vi "Sensor_Camera Auton Simple.vi"(7 "Final Task":T1(ring), 8 "error in":errorcluster, 9 "Second Drive Distance":dbl, 10 "First Turn Angle":dbl, 11 "First Drive Distance":dbl) -> (0 "error out":errorcluster)   [LabVIEW 2016]
uses:
  <vilib>/Rock Robotics/WPI/Gyro/WPI_GyroDevRef.ctl
  <vilib>/Rock Robotics/SystemInterfaces/AI/FPGA_AIChannel.ctl
  <vilib>/Rock Robotics/SystemInterfaces/spilib/spi_bus.ctl
  <vilib>/Rock Robotics/WPI/DriverStation/WPI_DriverStationAllianceInfo.ctl
  Vision/Vision Drive/Vision Drive.lvlib
  SubSystems/Drive/Drive System.lvlib
  SubSystems/Path Track/Path Track.lvlib
  SubSystems/Intake/Intake.lvlib
panel:
  in  "Vision Deadband":dbl=25.0 caption="Vision Deadband Distance (in.)"
  in  "Drive Magnitude":dbl format="%#_13g"
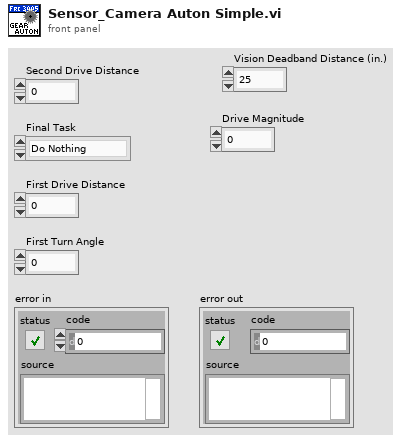
[diagram p1: front panel]
types:
  T1 = enum16{"Do Nothing", "Turn Up Field", "Turn to Boiler"}
  T2 = typedef "WPI_GyroDevRef.ctl" = cluster{"DevStatus":errorcluster, "Analog Channel":T3, "Offset":dbl, "Gain (VoltsPerDegree/Second)":dbl, "Gyro Type":enum16{"Analog", "XRS450"}, "Handle":i32, "SPI Bus":T4, "Device Found":bool, "Sample Rate":dbl, "Calibrate On Open":bool}
  T3 = typedef "FPGA_AIChannel.ctl" = enum8{"AI 0", "AI 1", "AI 2", "AI 3", "AI MXP 0", "AI MXP 1", "AI MXP 2", "AI MXP 3", "Invalid"}
  T4 = typedef "spi_bus.ctl" = enum16{"SPI On-Board, CS0", "SPI On-Board, CS1", "SPI On-Board, CS2", "SPI On-Board, CS3", "SPI MXP", "Invalid"}
  T5 = typedef "WPI_DriverStationAllianceInfo.ctl" = enum16{"Red", "Blue", "Invalid"}
  T6 = cluster{"Gyro":T2, "First Drive Distance":dbl, "First Turn Angle":dbl, "Alliance":T5, "Vision Timeout?":bool, "Vision Distance":dbl, "Second Drive Distance":dbl, "Final Task":enum16{"Do Nothing", "Turn Up Field", "Turn to Boiler"}, "Vision Angle":dbl}
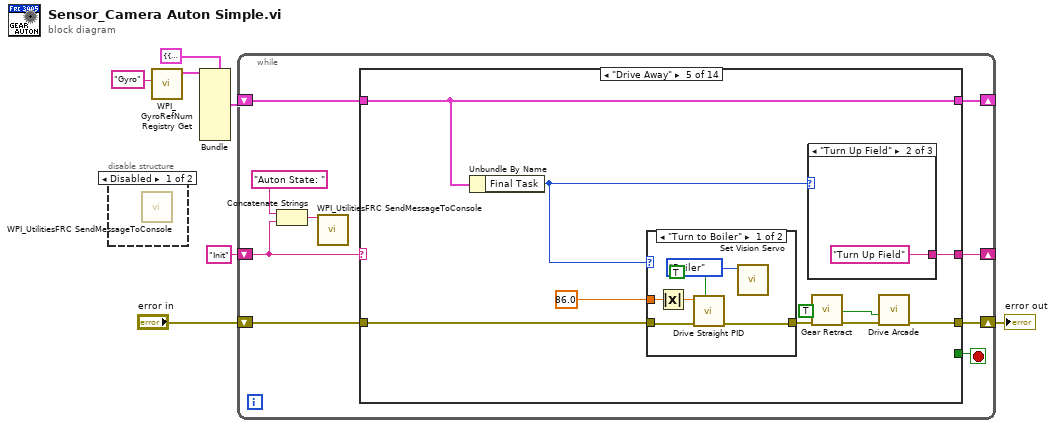
[diagram p0: block diagram]
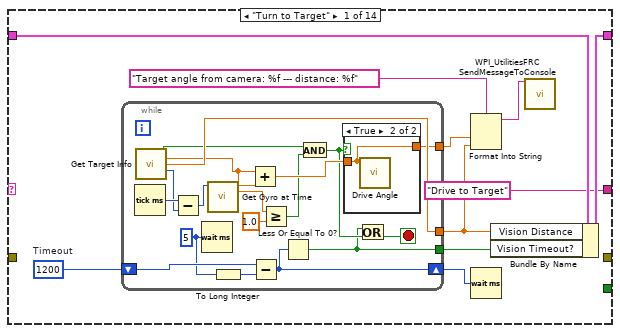
[diagram p3: hidden frame]
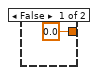
[diagram p4: hidden frame]
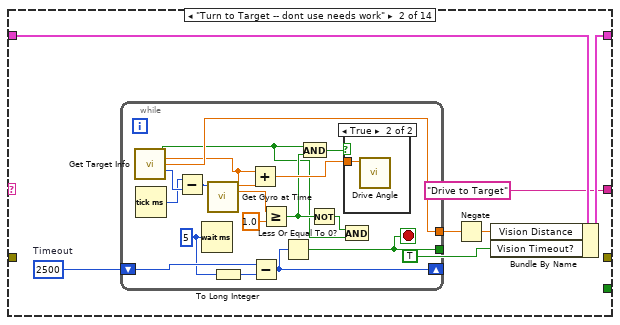
[diagram p5: hidden frame]
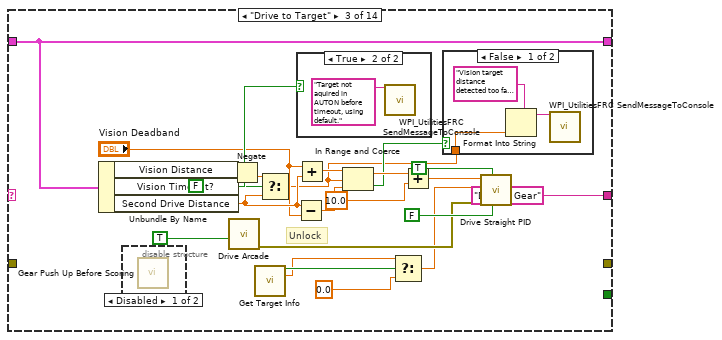
[diagram p7: hidden frame]
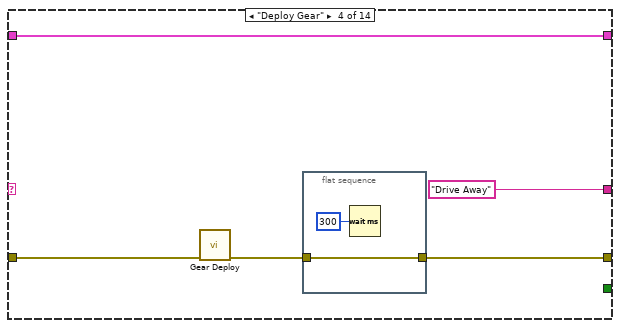
[diagram p11: hidden frame]
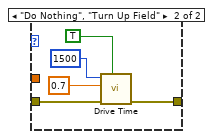
[diagram p12: hidden frame]
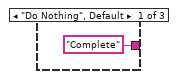
[diagram p13: hidden frame]
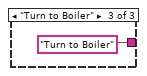
[diagram p14: hidden frame]
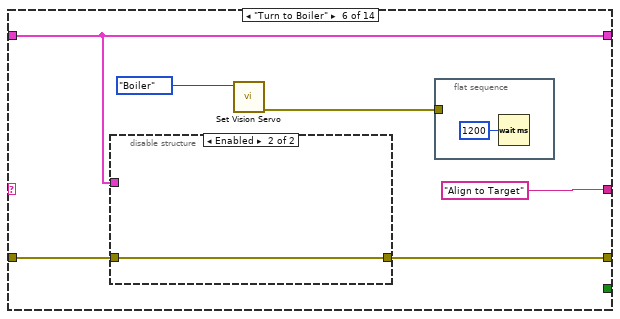
[diagram p15: hidden frame]
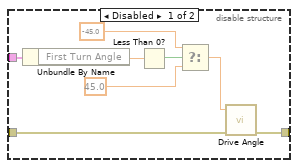
[diagram p16: hidden frame]
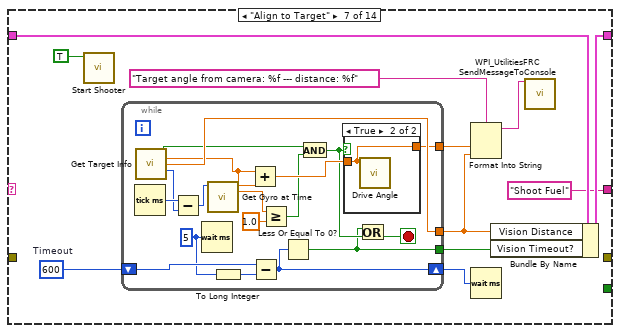
[diagram p17: hidden frame]
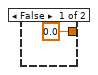
[diagram p18: hidden frame]
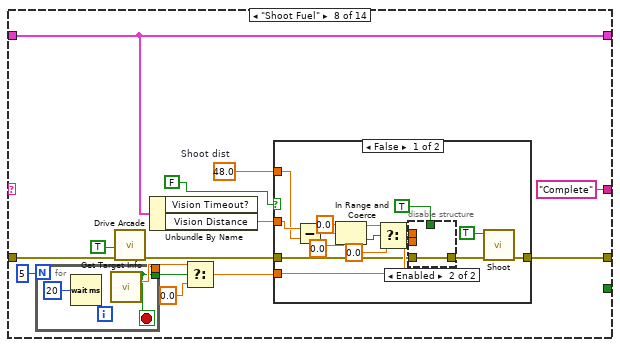
[diagram p19: hidden frame]
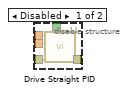
[diagram p20: hidden frame]
diagram:
  n1 = disable-structure shown="Disabled" {
    frame Disabled {
      n2 = call <vilib>:"WPI_UtilitiesFRC SendMessageToConsole.vi"() -> ()  [unwired: 15 in, 1 out]
    }
    frame Enabled {
    }
  }
  n3 = call <vilib>:"WPI_GyroRefNum Registry Get.vi"("refnum name"="Gyro") -> ("GyroDevRef"=w3:T2)  [unwired: 9 in, 1 out]
  n4 = Bundle(cluster=T6 {"Gyro"={"DevStatus"={"status"=FALSE, "code"=0, "source"=""}, "Analog Channel"=enum."AI 0", "Offset"=0.0, "Gain (VoltsPerDegree/Second)"=0.0, "Gyro Type"=enum."Analog", "Handle"=0, "SPI Bus"=enum."SPI On-Board, CS0", "Device Found"=FALSE, "Sample Rate"=0.0, "Calibrate On Open"=FALSE}, "First Drive Distance"=0.0, "First Turn Angle"=0.0, "Alliance"=enum."Red", "Vision Timeout?"=FALSE, "Vision Distance"=0.0, "Second Drive Distance"=0.0, "Final Task"=enum."Do Nothing", "Vision Angle"=0.0}, "Gyro"=w3) -> (w4:T6)  [unwired: 8 in]
  n5 = while {
    shift-right: [w14] -> _
    shift-left: "Init" -> [w10]
    shift-right: [w15] -> _
    shift-left: w4 -> [w16]
    shift-right: [w13] -> w7
    shift-left: "error in" -> [w12]
    stop <- w11 stop-if-true
    n6 = Concatenate Strings("Auton State: " ("string"), w10) -> (w8:string)
    n7 = call <vilib>:"WPI_UtilitiesFRC SendMessageToConsole.vi"("Message"=w8) -> ()  [unwired: 14 in, 1 out]
    n8 = case shown="\"Drive Away\"" w10 {
      selector: w10 -> [_ _ _ _ _ _ _ _ _ _ _ w241 _ _]
      tunnel: w16 -> [w26 w53 w75 w103 w107 w131 w155 w186 w223 w232 w236 w242 w255 w261]
      tunnel: [w24 w51 w75 w103 w107 w131 w153 w186 w223 w232 w236 w242 w250 w257] -> w15
      tunnel: ["Drive to Target" "Drive to Target" "Deploy Gear" ("refnum name") "Drive Away" ("refnum name") w112 "Align to Target" ("refnum name") "Shoot Fuel" "Complete" ("refnum name") "Drive Up Field" "Complete" "" "" "Drive Initial Distance and Turn" "Turn to Target"] -> w14
      tunnel: [_ _ _ w100 w110 w132 _ w187 w221 w227 _ _ w252 w259] -> w13
      tunnel: w12 -> [_ _ _ w101 w113 w133 _ w188 w222 w228 _ _ w251 w268]
      tunnel: [_ _ _ _ _ _ _ _ _ _ TRUE TRUE _ _] -> w11
      frame "Turn to Target" {
        w25 = 1200  # Timeout
        n9 = while {
          tunnel: [w40] -> w17
          shift-right: [w35] -> w22
          shift-left: w25 -> [w37]
          tunnel: [w31] -> w18
          tunnel: [w30] -> w21
          stop <- w32 stop-if-true
          w36 = u32 5 ("milliseconds to wait")
          n10 = Tick Count (ms)() -> (millisecond timer value=w29:u32)
          n11 = call "Get Target Info.vi"() -> ("Target Found?"=w38:bool, "Angle (deg)"=w39:dbl, "Distance (in)"=w40:dbl, "timestamp"=w28:u32)  [unwired: 11 in, 1 out]
          n12 = Subtract(x=w29, y=w28) -> (x-y=w27:u32)
          n13 = Wait (ms)(milliseconds to wait=w36) -> ()  [unwired: 1 out]
          n14 = call "Get Gyro at Time.vi"("Get ms ago"=w27) -> ("Angle"=w44:dbl)  [unwired: 9 in, 1 out]
          n15 = To Long Integer(number=w36) -> (32bit integer=w34:i32)
          n16 = Add(x=w39, y=w44) -> (x+y=w43:dbl)
          n17 = Subtract(x=w37, y=w34) -> (x-y=w35:i32)
          n18 = Greater Or Equal?(x=w39, y=1.0) -> (x >= y?=w41:bool)
          n19 = Less Or Equal To 0?(x=w35) -> (x <= 0?=w31:bool)
          n20 = And(x=w38, y=w41) -> (x .and. y?=w33:bool)
          n21 = case shown="True" w33 {
            tunnel: w43 -> [_ w46]
            tunnel: [0.0 w46] -> w30
            frame False {
            }
            frame True {
              n22 = call "Drive Angle.vi"("Angle"=w46) -> ()  [unwired: 10 in, 1 out]
            }
          }
          n23 = Or(x=w31, y=w33) -> (x .or. y?=w32:bool)
        }
        n24 = Format Into String(format string="Target angle from camera: %f --- distance: %f", w21, w17) -> (resulting string=w19:string)  [unwired: 2 in, 1 out]
        n25 = Wait (ms)(milliseconds to wait=w22) -> ()  [unwired: 1 out]
        n26 = Bundle By Name(cluster=w26, "Vision Distance"=w17, "Vision Timeout?"=w18) -> (w24:T6)
        n27 = call <vilib>:"WPI_UtilitiesFRC SendMessageToConsole.vi"("Message"=w19) -> ()  [unwired: 14 in, 1 out]
      }
      frame "Turn to Target -- dont use needs work" {
        w52 = 2500  # Timeout
        n28 = while {
          tunnel: [w66] -> w50
          shift-right: [w60] -> _
          shift-left: w52 -> [w62]
          tunnel: [w58] -> _
          stop <- w58 stop-if-true
          w61 = u32 5 ("milliseconds to wait")
          n29 = call "Get Target Info.vi"() -> ("Target Found?"=w63:bool, "Angle (deg)"=w65:dbl, "Distance (in)"=w66:dbl, "timestamp"=w56:u32)  [unwired: 11 in, 1 out]
          n30 = Tick Count (ms)() -> (millisecond timer value=w54:u32)
          n31 = Subtract(x=w54, y=w56) -> (x-y=w55:u32)
          n32 = Wait (ms)(milliseconds to wait=w61) -> ()  [unwired: 1 out]
          n33 = call "Get Gyro at Time.vi"("Get ms ago"=w55) -> ("Angle"=w70:dbl)  [unwired: 9 in, 1 out]
          n34 = To Long Integer(number=w61) -> (32bit integer=w59:i32)
          n35 = Add(x=w65, y=w70) -> (x+y=w69:dbl)
          n36 = Subtract(x=w62, y=w59) -> (x-y=w60:i32)
          n37 = Greater Or Equal?(x=w65, y=1.0) -> (x >= y?=w67:bool)
          n38 = Less Or Equal To 0?(x=w60) -> (x <= 0?=w58:bool)
          n39 = And(x=w63, y=w67) -> (x .and. y?=w57:bool)
          n40 = Not(x=w67) -> (.not. x?=w64:bool)
          n41 = And(x=w64, y=w63) -> ()  [unwired: 1 out]
          n42 = case shown="True" w57 {
            tunnel: w69 -> [_ w71]
            frame False {
            }
            frame True {
              n43 = call "Drive Angle.vi"("Angle"=w71) -> ()  [unwired: 10 in, 1 out]
            }
          }
        }
        n44 = Negate(x=w50) -> (-x=w48:dbl)
        n45 = Bundle By Name(cluster=w53, "Vision Distance"=w48, "Vision Timeout?"=TRUE) -> (w51:T6)
      }
      frame "Drive to Target" {
        # "Unlock"
        n46 = Unbundle By Name(w75) -> ("Vision Distance"=w89:dbl, "Vision Timeout?"=w87:bool, "Second Drive Distance"=w83:dbl)
        n47 = disable-structure shown="Disabled" {
          frame Disabled {
            n48 = call "Gear Push Up Before Scoring.vi"() -> ()  [unwired: 11 in, 1 out]
          }
          frame Enabled {
          }
        }
        n49 = call "Drive Arcade.vi"("Force? (F)"=TRUE) -> ("error out"=w90:errorcluster)  [unwired: 10 in]
        n50 = Negate(x=w89) -> (-x=w72:dbl)
        n51 = call "Get Target Info.vi"() -> ("Target Found?"=w77:bool, "Angle (deg)"=w74:dbl)  [unwired: 11 in, 3 out]
        n52 = Select(t=w72, s=FALSE, f=w83) -> (s? t:f=w80:dbl)
        n53 = Subtract(x=w83, y="Vision Deadband") -> (x-y=w85:dbl)
        n54 = case shown="True" w87 {
          frame False {
          }
          frame True {
            n55 = call <vilib>:"WPI_UtilitiesFRC SendMessageToConsole.vi"("Message"="Target not aquired in AUTON before timeout, using default.") -> ()  [unwired: 14 in, 1 out]
          }
        }
        n56 = Add(x="Vision Deadband", y=w83) -> (x+y=w84:dbl)
        n57 = In Range and Coerce(upper limit=w84, x=w80, lower limit=w85) -> (coerced(x)=w86:dbl, In Range?=w81:bool)
        n58 = Select(t=w74, s=w77, f=0.0 ("Peg dist")) -> (s? t:f=w73:dbl)
        n59 = Add(x=w86, y=10.0 ("Peg dist")) -> (x+y=w78:dbl)
        n60 = case shown="False" w81 {
          tunnel: w80 -> [w96 _]
          frame False {
            n61 = Format Into String(format string="Vision target distance detected too far! Recieved %f" ("Message"), w96) -> (resulting string=w95:string)  [unwired: 2 in, 1 out]
            n62 = call <vilib>:"WPI_UtilitiesFRC SendMessageToConsole.vi"("Message"=w95) -> ()  [unwired: 14 in, 1 out]
          }
          frame True {
          }
        }
        n63 = call "Drive Straight PID.vi"("Force? (F)"=FALSE, "Wait for Completion? (F)"=TRUE, "error in"=w90, "angle offset (0)"=w73, "Distance (in)"=w78) -> ()  [unwired: 6 in, 1 out]
      }
      frame "Deploy Gear" {
        n64 = call "Gear Deploy.vi"("error in"=w101) -> ("error out"=w102:errorcluster)  [unwired: 10 in]
        n65 = flat-sequence {
          tunnel: w102 -> [w105]
          tunnel: [w105] -> w100
          frame #0 {
            n66 = Wait (ms)(milliseconds to wait=u32 300) -> ()  [unwired: 1 out]
          }
        }
      }
      frame "Drive Away" {
        n67 = Unbundle By Name(w107) -> ("Final Task"=w108:T1)
        n68 = case shown="\"Turn to Boiler\"" w108 {
          tunnel: [w119 w125] -> w114
          tunnel: w113 -> [w120 w124]
          tunnel: 86.0 -> [w118 _]
          frame "Turn to Boiler" {
            n69 = Absolute Value(x=w118) -> (abs(x)=w117:dbl)
            n70 = call "Drive Straight PID.vi"("Wait for Completion? (F)"=TRUE, "error in"=w120, "Distance (in)"=w117) -> ("error out"=w119:errorcluster)  [unwired: 8 in]
            n71 = call "Set Vision Servo.vi"("Setting"=enum16{"Custom", "Boiler", "Gear"}."Boiler") -> ()  [unwired: 10 in, 1 out]
          }
          frame "Do Nothing", "Turn Up Field" {
            n72 = call "Drive Time.vi"("Wait for Completion? (F)"=TRUE, "error in"=w124, "Y Axis"=0.7, "Time (ms)"=u32 1500) -> ("error out"=w125:errorcluster)  [unwired: 7 in]
          }
        }
        n73 = case shown="\"Turn Up Field\"" w108 {
          tunnel: ["Complete" ("refnum name") "Turn Up Field" ("refnum name") "Turn to Boiler" ("refnum name")] -> w112
          frame "Do Nothing", Default {
          }
          frame "Turn Up Field" {
          }
          frame "Turn to Boiler" {
          }
        }
        n74 = call "Gear Retract.vi"("error in"=w114) -> ("error out"=w111:errorcluster)  [unwired: 10 in]
        n75 = call "Drive Arcade.vi"("error in"=w111, "Force? (F)"=TRUE) -> ("error out"=w110:errorcluster)  [unwired: 9 in]
      }
      frame "Turn to Boiler" {
        n76 = disable-structure shown="Enabled" {
          disable-tunnel: w133 -> [w142 w143]
          disable-tunnel: [w141 w143] -> w132
          disable-tunnel: w131 -> [w140 _]
          frame Disabled {
            n77 = Unbundle By Name(w140) -> ("First Turn Angle"=w139:dbl)
            n78 = Less Than 0?(x=w139) -> (x < 0?=w138:bool)
            n79 = Select(t=-45.0 ("Angle"), s=w138, f=45.0 ("Angle")) -> (s? t:f=w135:dbl)
            n80 = call "Drive Angle.vi"("error in"=w142, "Angle"=w135) -> ("error out"=w141:errorcluster)  [unwired: 9 in]
          }
          frame Enabled {
          }
        }
        n81 = call "Set Vision Servo.vi"("Setting"=enum16{"Custom", "Boiler", "Gear"}."Boiler") -> ("error out"=w129:errorcluster)  [unwired: 10 in]
        n82 = flat-sequence {
          tunnel: w129 -> [_]
          frame #0 {
            n83 = Wait (ms)(milliseconds to wait=u32 1200) -> ()  [unwired: 1 out]
          }
        }
      }
      frame "Align to Target" {
        w154 = 600  # Timeout
        n84 = call "Start Shooter.vi"("Enabled? (F)"=TRUE) -> ()  [unwired: 10 in, 1 out]
        n85 = while {
          tunnel: [w169] -> w146
          shift-right: [w164] -> w151
          shift-left: w154 -> [w166]
          tunnel: [w160] -> w147
          tunnel: [w159] -> w150
          stop <- w161 stop-if-true
          w165 = u32 5 ("milliseconds to wait")
          n86 = Tick Count (ms)() -> (millisecond timer value=w158:u32)
          n87 = call "Get Target Info.vi"() -> ("Target Found?"=w167:bool, "Angle (deg)"=w168:dbl, "Distance (in)"=w169:dbl, "timestamp"=w157:u32)  [unwired: 11 in, 1 out]
          n88 = Subtract(x=w158, y=w157) -> (x-y=w156:u32)
          n89 = Wait (ms)(milliseconds to wait=w165) -> ()  [unwired: 1 out]
          n90 = call "Get Gyro at Time.vi"("Get ms ago"=w156) -> ("Angle"=w173:dbl)  [unwired: 9 in, 1 out]
          n91 = To Long Integer(number=w165) -> (32bit integer=w163:i32)
          n92 = Add(x=w168, y=w173) -> (x+y=w172:dbl)
          n93 = Subtract(x=w166, y=w163) -> (x-y=w164:i32)
          n94 = Greater Or Equal?(x=w168, y=1.0) -> (x >= y?=w170:bool)
          n95 = Less Or Equal To 0?(x=w164) -> (x <= 0?=w160:bool)
          n96 = And(x=w167, y=w170) -> (x .and. y?=w162:bool)
          n97 = case shown="True" w162 {
            tunnel: w172 -> [_ w175]
            tunnel: [0.0 w175] -> w159
            frame False {
            }
            frame True {
              n98 = call "Drive Angle.vi"("Angle"=w175) -> ()  [unwired: 10 in, 1 out]
            }
          }
          n99 = Or(x=w160, y=w162) -> (x .or. y?=w161:bool)
        }
        n100 = Format Into String(format string="Target angle from camera: %f --- distance: %f", w150, w146) -> (resulting string=w148:string)  [unwired: 2 in, 1 out]
        n101 = Wait (ms)(milliseconds to wait=w151) -> ()  [unwired: 1 out]
        n102 = Bundle By Name(cluster=w155, "Vision Distance"=w146, "Vision Timeout?"=w147) -> (w153:T6)
        n103 = call <vilib>:"WPI_UtilitiesFRC SendMessageToConsole.vi"("Message"=w148) -> ()  [unwired: 14 in, 1 out]
      }
      frame "Shoot Fuel" {
        w178 = 48.0  # Shoot dist
        n104 = for {
          N: 5 -> [_]
          tunnel: [w191] -> w185
          tunnel: [w192] -> w183
          stop <- w191 stop-if-true
          n105 = Wait (ms)(milliseconds to wait=u32 20) -> ()  [unwired: 1 out]
          n106 = call "Get Target Info.vi"() -> ("Target Found?"=w191:bool, "Angle (deg)"=w192:dbl)  [unwired: 11 in, 3 out]
        }
        n107 = call "Drive Arcade.vi"("error in"=w188, "Force? (F)"=TRUE) -> ("error out"=w180:errorcluster)  [unwired: 9 in]
        n108 = Unbundle By Name(w186) -> ("Vision Distance"=w181:dbl)  [unwired: 1 out]
        n109 = Select(t=w183, s=w185, f=0.0 ("Peg dist")) -> (s? t:f=w182:dbl)
        n110 = case shown="False" FALSE {
          tunnel: [w206 w216] -> w187
          tunnel: w182 -> [w204 _]
          tunnel: w181 -> [w201 _]
          tunnel: w180 -> [w202 w215]
          tunnel: w178 -> [w200 _]
          frame False {
            n111 = Subtract(x=w201, y=w200) -> (x-y=w199:dbl)
            n112 = In Range and Coerce(upper limit=0.0, x=w199, lower limit=0.0) -> (coerced(x)=w194:dbl, In Range?=w195:bool)
            n113 = Select(t=w194, s=w195, f=0.0) -> (s? t:f=w196:dbl)
            n114 = disable-structure shown="Enabled" {
              disable-tunnel: [w212 w213] -> w205
              disable-tunnel: w204 -> [w211 _]
              disable-tunnel: TRUE ("Wait for Completion? (F)") -> [w210 _]
              disable-tunnel: w202 -> [w209 w213]
              disable-tunnel: w196 -> [w208 _]
              frame Disabled {
                n115 = call "Drive Straight PID.vi"("Wait for Completion? (F)"=w210, "error in"=w209, "angle offset (0)"=w211, "Distance (in)"=w208) -> ("error out"=w212:errorcluster)  [unwired: 7 in]
              }
              frame Enabled {
              }
            }
            n116 = call "Shoot.vi"("error in"=w205, "Enabled? (F)"=TRUE) -> ("error out"=w206:errorcluster)  [unwired: 9 in]
          }
          frame True {
            n117 = call <vilib>:"WPI_UtilitiesFRC SendMessageToConsole.vi"("Message"="Boiler not found! Fuel will not be shot at this time.", "error in (no error)"=w215) -> ("error out"=w216:errorcluster)  [unwired: 13 in]
          }
        }
      }
      frame "Turn Up Field" {
        n118 = call "Drive Angle.vi"("error in"=w222, "Drive Magnitude"="Drive Magnitude", "Angle"=0.0) -> ("error out"=w221:errorcluster)  [unwired: 8 in]
        n119 = Wait (ms)(milliseconds to wait=u32 1200) -> ()  [unwired: 1 out]
      }
      frame "Drive Up Field" {
        n120 = call "Drive Arcade.vi"("error in"=w228, "Force? (F)"=TRUE) -> ("error out"=w225:errorcluster)  [unwired: 9 in]
        n121 = call "Drive Straight PID.vi"("Force? (F)"=FALSE, "Wait for Completion? (F)"=TRUE, "error in"=w225, "Distance (in)"=-100.0) -> ("error out"=w227:errorcluster)  [unwired: 7 in]
      }
      frame "Complete" {
        n122 = call <vilib>:"WPI_UtilitiesFRC SendMessageToConsole.vi"("Message"="Auton routine complete") -> ()  [unwired: 14 in, 1 out]
      }
      frame "", Default {
        n123 = Concatenate Strings("Invalid State Reached Auton: " ("string"), w241) -> (w239:string)
        n124 = call <vilib>:"WPI_UtilitiesFRC SendMessageToConsole.vi"("Message"=w239) -> ()  [unwired: 14 in, 1 out]
      }
      frame "Init" {
        n125 = Unbundle By Name(w255) -> ("Gyro"=w254:T2)
        n126 = call <vilib>:"WPI_GyroReset.vi"("error in"=w251, "GyroDevRef"=w254) -> ("error out"=w252:errorcluster)  [unwired: 8 in, 1 out]
        n127 = call <vilib>:"WPI_DriverStationGet Alliance Info.vi"() -> ("Alliance"=w245:T5)  [unwired: 10 in, 1 out]
        n128 = Bundle By Name(cluster=w255, "First Drive Distance"="First Drive Distance", "First Turn Angle"="First Turn Angle", "Alliance"=w245, "Final Task"="Final Task", "Second Drive Distance"="Second Drive Distance") -> (w250:T6)
        n129 = Format Into String(format string="AutoReported Alliance: %s " ("Message"), w245) -> (resulting string=w243:string)  [unwired: 2 in, 1 out]
        n130 = call <vilib>:"WPI_UtilitiesFRC SendMessageToConsole.vi"("Message"=w243) -> ()  [unwired: 14 in, 1 out]
      }
      frame "Drive Initial Distance and Turn" {
        n131 = Unbundle By Name(w261) -> ("First Turn Angle"=w263:dbl, "Alliance"=w266:T5)
        n132 = Unbundle By Name(w261) -> ("First Drive Distance"=w258:dbl)
        n133 = Equal?(x=w266, y=WPI_DriverStationAllianceInfo."Blue") -> (x = y?=w264:bool)
        n134 = Negate(x=w263) -> (-x=w262:dbl)
        n135 = call "Drive Straight PID.vi"("Wait for Completion? (F)"=TRUE, "error in"=w268, "Distance (in)"=w258) -> ("error out"=w269:errorcluster)  [unwired: 8 in]
        n136 = Select(t=w263, s=w264, f=w262) -> (s? t:f=w256:dbl)
        n137 = call "Drive Angle.vi"("error in"=w269, "Drive Magnitude"=0.0, "Angle"=w256) -> ("error out"=w259:errorcluster)  [unwired: 8 in]
        n138 = Bundle By Name(cluster=w261, "First Turn Angle"=w256) -> (w257:T6)
        n139 = flat-sequence {
          tunnel: w259 -> [_]
          frame #0 {
            n140 = Wait (ms)(milliseconds to wait=u32 400) -> ()  [unwired: 1 out]
          }
        }
      }
    }
  }
  "error out" <- w7
